vi "PH_Powermeter_BaseClass.panel.vi"(0 "object ref":refnum<vi>, 5 "error in (no error)":errorcluster) -> (19 "error out":errorcluster)   [LabVIEW 2014, in "PH_Powermeter_BaseClass.lvlib"]
doc: "By this VI apowermeter can be operated. \n\nThe panel is divided into the Tab Control which contains three pages and the most important elements.\nThe 1st page of the Tab Control contains the general information Range, Trigger Level, Scaling Factor (the user can set these values), Uncorrected Value and Serial Number (these are indicators). \nThe 2nd page contains everything relevant for the Statistics Mode of the powermeter. Here you can Start/Stop the statistic data collection, set the Number of Pulses, Percentage of Pulses and the Number of Samples. The Cluster 'Statistic Data' views the evaluated statistic data.\nThe 3rd page contains the rarely needed status-information of the powermeter. The string views data like Active Sensitivity, Offset, Resolution and so on.\n\nBelow the Tab Control you can see: \n - Current Value views the value that is currently being displayed on the device's screen. The correct unit is appended.\n - Powermeter views the Device State: blue means no info\n darkgreen means off\n lightgreen means operating\n yellow means error detected\n - EXIT closes the front panel (GUI), while\n - Delete Instance disconnects and removes the instance from the PCS.\n\n\nLicense Agreement for this software:\n\nCopyright (C)\nGesellschaft für Schwerionenforschung, GSI\nPlanckstr. 1\n64291 Darmstadt\nGermany\n\nContact: D.Beck@gsi.de \n\nThis program is free software; you can redistribute it and/or modify it under the terms of the GNU General Public License as published by the Free Software Foundation; either version 2 of the license, or (at your option) any later version.\n\nThis program is distributed in the hope that it will be useful, but WITHOUT ANYW ARRANTY; without even the implied warranty of MERCHANTABILITY or FITNESS FOR A PARTICULAR PURPOSE. See the GNU General License for more details (http://www.gnu.org).\n\nGesellschaft für Schwerionenforschung, GSI\nPlanckstr. 1, 64291 Darmstadt, Germany\nFor all questions and ideas contact: M.Richter@gsi.de, H.Brand@gsi.de or D.Beck@gsi.de.\nLast update: 18-DEC-2002"
uses:
  PH_Powermeter_BaseClass.lvlib
  PH_StatusHandler/PH_StatusHandler.GUI element.ctl
  PH_Powermeter_BaseClass.Connection.ctl
  PH_Powermeter_BaseClass.State.ctl
  PH_Powermeter_BaseClass.Head Attributes.ctl
  PH_Powermeter_BaseClass.Energy.ctl
  PH_gentec_BaseClass.Head Settings.ctl
  PH_Powermeter_BaseClass.GUI Refs.ctl
  CS_Core/CSObj/CSObj.lvlib
  PH_Common/PH_Common.lvlib
  PH_Class/PH_Class.lvlib
  CS_Core/CSSystem/CSSystemLib/CSSystemLib.lvlib
  PH_StatusHandler/PH_StatusHandler.lvlib
panel:
  in  "Tab Control":enum32{"Main", "Sets", "Information"}(tab)
  in  "Wavelength":u32=1 caption="nm"
  in  "Trigger Level":dbl caption="%"
  in  "Range":u32(ring) items=["Scale 1", "Scale 2", "Scale 3"]
  in  "Scaling Factor":dbl=1.0
  out "Energy evolution":dbl(graph)
  out "Energy":T1={"current Value"=-1.0, "unscaled"=0.0, "Scaling Factor"=1.0} {"unscaled" format="%#_6p"; "current Value" format="%#.1p"}
  out "Current Settings":T2={"Trigger Level"=0.0, "Wavelength"=1, "Range"=0}
  out "Wanted Settings":T2={"Trigger Level"=0.0, "Wavelength"=1, "Range"=0}
  out "VISA resource":refnum<visa-resource-name>
  out "Connection":T3
  out "Head Attributes":T5={"Instrument Type"="---", "Head Version"="---", "Head Name"="---", "Serial Number"="---", "Firmware"="---", "Sensor Type"="---", "MinimumRange"=0, "Maximum Range"=0, "Min Wavelength"=-1, "Max Wavelength"=-1}
  out "PSDB Status":u32(colorbox)=6618880 caption="PSDB"
  out "Status":T6 caption="Powermeter"
  in  "Delete":bool
  in  "Exit":bool
  # "PCS"
  # "3.40"
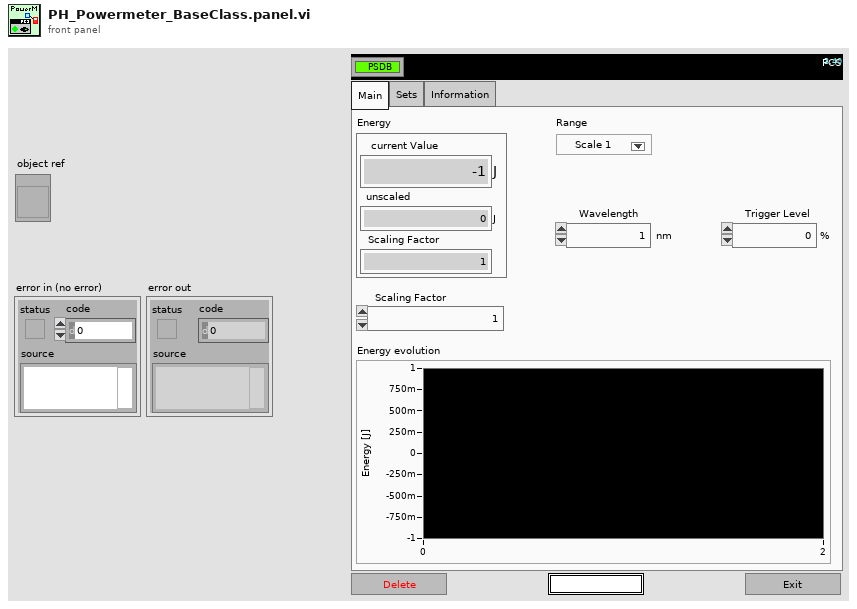
[diagram p1: front panel]
types:
  T1 = typedef "PH_Powermeter_BaseClass.lvlib/PH_Powermeter_BaseClass.Energy.ctl" = cluster{"current Value":dbl, "unscaled":dbl, "Scaling Factor":dbl}
  T2 = typedef "PH_Powermeter_BaseClass.lvlib/PH_gentec_BaseClass.Head Settings.ctl" = cluster{"Trigger Level":dbl, "Wavelength":u32, "Range":u32}
  T3 = typedef "PH_Powermeter_BaseClass.lvlib/PH_Powermeter_BaseClass.Connection.ctl" = cluster{"failed checks":i8, "Timeout":bool, "Data read":string, "Failure":bool, "Error":bool, "State":T4}
  T4 = typedef "PH_Powermeter_BaseClass.lvlib/PH_Powermeter_BaseClass.State.ctl" = enum32{"off", "operating", "opened", "checked", "connected", "Sets to change", "running"}
  T5 = typedef "PH_Powermeter_BaseClass.lvlib/PH_Powermeter_BaseClass.Head Attributes.ctl" = cluster{"Instrument Type":string, "Head Version":string, "Head Name":string, "Serial Number":string, "Firmware":string, "Sensor Type":string, "MinimumRange":u32, "Maximum Range":u32, "Min Wavelength":i32, "Max Wavelength":i32}
  T6 = typedef "PH_StatusHandler.lvlib/PH_StatusHandler.GUI element.ctl" = u16
  T7 = typedef "PH_Powermeter_BaseClass.lvlib/PH_Powermeter_BaseClass.GUI Refs.ctl" = cluster{"Head Attributes":refnum<vi>, "Energy":refnum<vi>, "Connection":refnum<vi>, "VISA Resource":refnum<vi>, "Energy evolution":refnum<vi>, "Scaling Factor":refnum<vi>, "Range":refnum<vi>, "Wavelength":refnum<vi>, "Trigger Level":refnum<vi>, "Wanted Settings":refnum<vi>, "Current Settings":refnum<vi>}
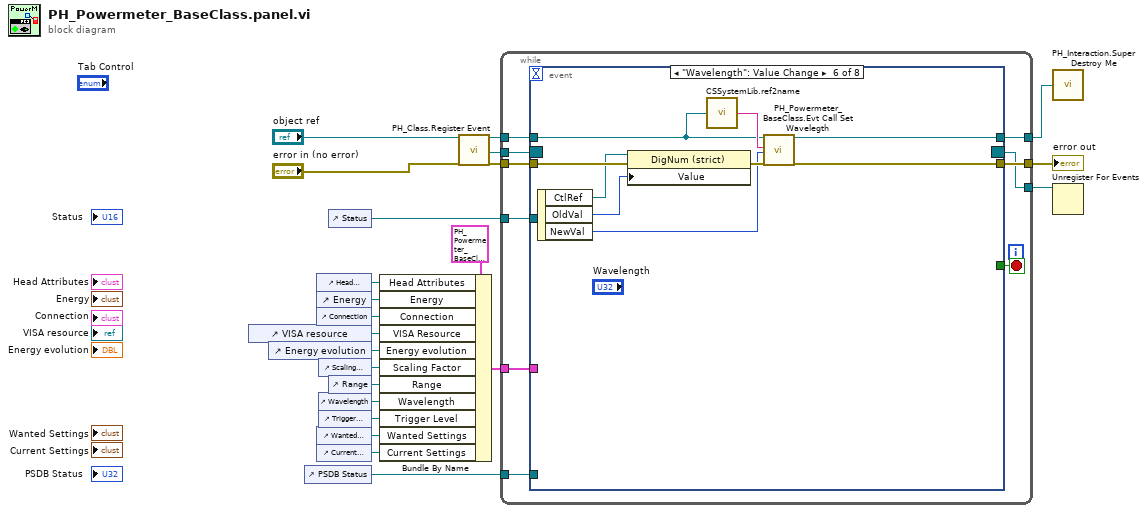
[diagram p0: block diagram]
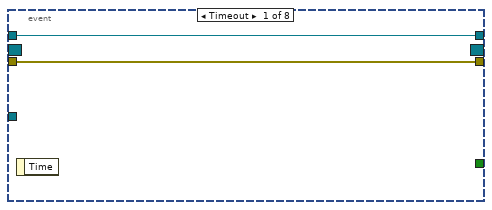
[diagram p2: hidden frame]
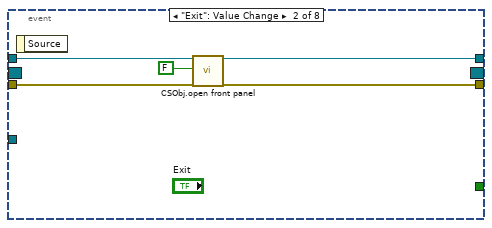
[diagram p3: hidden frame]
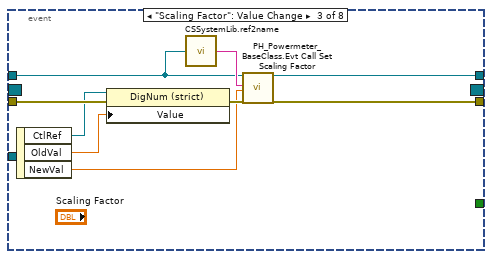
[diagram p4: hidden frame]
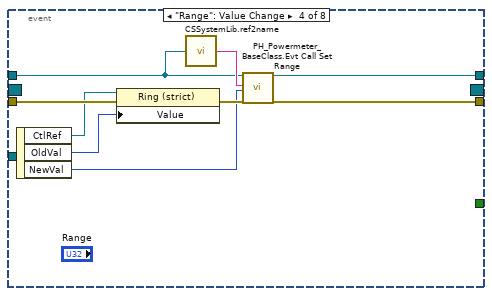
[diagram p5: hidden frame]
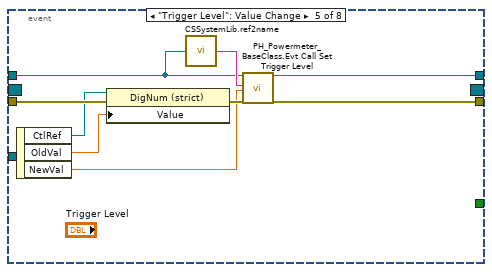
[diagram p6: hidden frame]
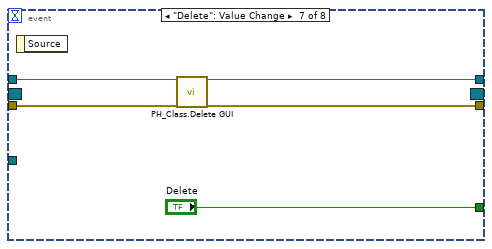
[diagram p7: hidden frame]
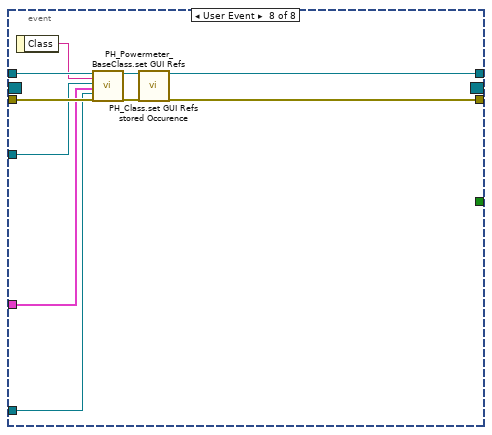
[diagram p8: hidden frame]
diagram:
  n1 = control-ref of="VISA resource"() -> (w9:refnum<vi>)
  n2 = control-ref of="Energy evolution"() -> (w8:refnum<vi>)
  n3 = control-ref of="PSDB Status"() -> (w16:refnum<vi>)
  n4 = control-ref of="Head Attributes"() -> (w3:refnum<vi>)
  n5 = control-ref of="Energy"() -> (w12:refnum<vi>)
  n6 = control-ref of="Connection"() -> (w11:refnum<vi>)
  n7 = control-ref of="Wanted Settings"() -> (w1:refnum<vi>)
  n8 = control-ref of="Current Settings"() -> (w2:refnum<vi>)
  n9 = control-ref of="Scaling Factor"() -> (w7:refnum<vi>)
  n10 = control-ref of="Wavelength"() -> (w5:refnum<vi>)
  n11 = control-ref of="Trigger Level"() -> (w4:refnum<vi>)
  n12 = control-ref of="Status"() -> (w17:refnum<vi>)
  n13 = control-ref of="Range"() -> (w6:refnum<vi>)
  n14 = Bundle By Name(cluster=T7 {"Head Attributes"=refnum, "Energy"=refnum, "Connection"=refnum, "VISA Resource"=refnum, "Energy evolution"=refnum, "Scaling Factor"=refnum, "Range"=refnum, "Wavelength"=refnum, "Trigger Level"=refnum, "Wanted Settings"=refnum, "Current Settings"=refnum} ("GUI References"), "Head Attributes"=w3, "Energy"=w12, "Connection"=w11, "VISA Resource"=w9, "Energy evolution"=w8, "Scaling Factor"=w7, "Range"=w6, "Wavelength"=w5, "Trigger Level"=w4, "Wanted Settings"=w1, "Current Settings"=w2) -> (w10:T7)
  n15 = call "PH_Class.Register Event.vi"("i ref in"="object ref", "error in (no error)"="error in (no error)") -> ("i ref out"=w21:refnum<vi>, "Event Registration Refnum"=w19:refnum<event-registration>, "error out"=w20:errorcluster)  [unwired: 15 in]
  n16 = while {
    tunnel: w21 -> [w30]
    tunnel: [w29] -> w22
    tunnel: w20 -> [w32]
    tunnel: [w31] -> w23
    tunnel: w19 -> [w28]
    tunnel: [w27] -> w18
    tunnel: w17 -> [w26]
    tunnel: w16 -> [w25]
    tunnel: w10 -> [w24]
    stop <- w33 stop-if-true
    n17 = event shown="[5] \"Wavelength\": Value Change" {
      selector: w28 -> [_ _ _ _ _ _ _ _]
      dyn-events: [_ _ _ _ _ _ _ _] -> w27
      timeout: _ -> [_ _ _ _ _ _ _ _]
      tunnel: [_ _ _ _ _ _ "Delete" _] -> w33
      tunnel: w30 -> [w34 w40 w47 w56 w65 w74 w79 w91]
      tunnel: w32 -> [w35 w38 w45 w54 w63 w72 w80 w90]
      tunnel: [w35 w37 w44 w53 w62 w71 w77 w83] -> w31
      tunnel: [w34 w36 w46 w55 w64 w73 w78 w84] -> w29
      tunnel: w26 -> [_ _ _ _ _ _ _ w89]
      tunnel: w25 -> [_ _ _ _ _ _ _ w87]
      tunnel: w24 -> [_ _ _ _ _ _ _ w82]
      event Timeout {
        n18 = event-data() -> ()  [unwired: 1 in, 1 out]
      }
      event "Exit": Value Change {
        n19 = event-data() -> ()  [unwired: 1 in, 1 out]
        n20 = call "CSObj.open front panel.vi"("i ref in"=w40, "frontPanelOpen"=FALSE ("front panel open"), "error in (no error)"=w38) -> ("i ref out"=w36:refnum<vi>, "error out"=w37:errorcluster)  [unwired: 15 in]
      }
      event "Scaling Factor": Value Change {
        n21 = event-data() -> ("CtlRef"=w43:refnum<vi>, "OldVal"=w42:dbl, "NewVal"=w41:dbl)  [unwired: 1 in]
        n22 = property class="DigNum (strict)"(reference=w43, error in=w45, "Value"=w42) -> (error out=w48:errorcluster)  [unwired: 1 out]
        n23 = call "CSSystemLib.ref2name.vi"("obj refnum"=w47) -> ("name"=w49:string)
        n24 = call "PH_Powermeter_BaseClass.Evt Call Set Scaling Factor.vi"("i ref in"=w47, "Instance"=w49, "Scaling Factor"=w41, "error in (no error)"=w48) -> ("i ref out"=w46:refnum<vi>, "error out"=w44:errorcluster)  [unwired: 14 in]
      }
      event "Range": Value Change {
        n25 = event-data() -> ("CtlRef"=w52:refnum<vi>, "OldVal"=w51:u32, "NewVal"=w50:u32)  [unwired: 1 in]
        n26 = property class="Ring (strict)"(reference=w52, error in=w54, "Value"=w51) -> (error out=w57:errorcluster)  [unwired: 1 out]
        n27 = call "CSSystemLib.ref2name.vi"("obj refnum"=w56) -> ("name"=w58:string)
        n28 = call "PH_Powermeter_BaseClass.Evt Call Set Range.vi"("i ref in"=w56, "Instance"=w58, "Range"=w50, "error in (no error)"=w57) -> ("i ref out"=w55:refnum<vi>, "error out"=w53:errorcluster)  [unwired: 14 in]
      }
      event "Trigger Level": Value Change {
        n29 = event-data() -> ("CtlRef"=w61:refnum<vi>, "OldVal"=w60:dbl, "NewVal"=w59:dbl)  [unwired: 1 in]
        n30 = property class="DigNum (strict)"(reference=w61, error in=w63, "Value"=w60) -> (error out=w66:errorcluster)  [unwired: 1 out]
        n31 = call "CSSystemLib.ref2name.vi"("obj refnum"=w65) -> ("name"=w67:string)
        n32 = call "PH_Powermeter_BaseClass.Evt Call Set Trigger Level.vi"("i ref in"=w65, "Instance"=w67, "Scaling Factor"=w59, "error in (no error)"=w66) -> ("i ref out"=w64:refnum<vi>, "error out"=w62:errorcluster)  [unwired: 14 in]
      }
      event "Wavelength": Value Change {
        n33 = event-data() -> ("CtlRef"=w70:refnum<vi>, "OldVal"=w69:u32, "NewVal"=w68:u32)  [unwired: 1 in]
        n34 = property class="DigNum (strict)"(reference=w70, error in=w72, "Value"=w69) -> (error out=w75:errorcluster)  [unwired: 1 out]
        n35 = call "CSSystemLib.ref2name.vi"("obj refnum"=w74) -> ("name"=w76:string)
        n36 = call "PH_Powermeter_BaseClass.Evt Call Set Wavelegth.vi"("i ref in"=w74, "Instance"=w76, "Scaling Factor"=w68, "error in (no error)"=w75) -> ("i ref out"=w73:refnum<vi>, "error out"=w71:errorcluster)  [unwired: 14 in]
      }
      event "Delete": Value Change {
        n37 = event-data() -> ()  [unwired: 1 in, 1 out]
        n38 = call "PH_Class.Delete GUI.vi"("VI in"=w79, "error in (no error)"=w80) -> ("VI out"=w78:refnum<vi>, "error out"=w77:errorcluster)  [unwired: 16 in]
      }
      event User Event {
        n39 = event-data() -> ("Class"=w88:string)  [unwired: 1 in]
        n40 = call "PH_Powermeter_BaseClass.set GUI Refs.vi"("VI in"=w91, "Class"=w88, "Status GUI Reference"=w89, "Powermeter Base Class GUI References"=w82, "PSDB Status GUI Reference"=w87, "error in (no error)"=w90) -> ("VI out"=w86:refnum<vi>, "error out"=w85:errorcluster)  [unwired: 12 in]
        n41 = call "PH_Class.set GUI Refs stored Occurence.vi"("i ref in"=w86, "error in (no error)"=w85) -> ("i ref out"=w84:refnum<vi>, "error out"=w83:errorcluster)  [unwired: 16 in]
      }
    }
  }
  "error out" <- w23
  n42 = call "PH_Interaction.Super Destroy Me.vi"("i ref out"=w22) -> ()
  n43 = Unregister For Events(event registration refnum=w18) -> ()  [unwired: 1 in, 1 out]
